vi "single sweep - next chunk - V2-2.vi"(4 "algorithm":string="statemachine", 5 "cursor bracket: Scan, win":refnum<vi>, 6 "mode":enum16{"first time", "uniform", "adaptive"}(ring)=enum."adaptive", 7 "Plot:response":refnum<vi>, 9 "x + iy":cdb[](array[numeric])=[0.0014961444378751654-0.005494848789731022i, 0.0014279223595474386-0.005470747752736027i, 0.001513711413730512-0.00552874878044623i, 0.001502407562898675-0.005445638194888334i, 0.0015845696982058808-0.005437153149732619i, 0.0015101628497750257-0.005522728337901211i, 0.0015131031857027845-0.005520920485579818i, 0.0015751707865244427-0.005432155579139866i, 0.001381283887581937-0.0055376532176146485i, 0.0013869914972504977-0.005471269712968517i], 10 "chunks":T1={"start F"=1400000.0, "stop F"=3000000.0, "total number of points"=6000, "chunk size"=10, "freq step (Hz)"=400.0, "update rate (Hz)"=250.0, "adaptive parameters"={"wavepacket"={"R"=0.5, "wave number"=15.0, "delta k"=7.0, "radii vector"=[], "radial section"=[], "wave vector"=22.0, "wavepacket is"=TRUE}, "number of grid points"=50, "decimation threshold"=1, "Voltage range"=0.1, "target freq step"=20.0, "target spot size"=0.05, "factor"=1.0, "another factor"=1.0, "analyze last # sec"=1, "scale factor"=10}, "total sweep time (sec)"=24.0, "chunk time (sec)"=0.04, "spot size (V)"=5.8152639158694506e-05, "uniform freq step (Hz)"=266.6666666666667, "next start freq"=1412960.0000000002} {"next start freq" format="%#_4f"; "uniform freq step (Hz)" format="%#_3f"; "spot size (V)" format="%#_2f"; "adaptive parameters"."wavepacket"."delta k" format="%#_3f"; "adaptive parameters"."wavepacket"."wave number" format="%#_3f"; "adaptive parameters"."wavepacket"."R" format="%#_3f"; "freq step (Hz)" format="%#_2f"; "stop F" format="%#_3f"; "start F" format="%#_3f"}, 11 "F Array in":dbl[](array[numeric])=[1408640.0000000002, 1408672.0000000002, 1408704.0000000002, 1408736.0000000002, 1408768.0000000002, 1408800.0000000002, 1408832.0000000002, 1408864.0000000002, 1408896.0000000002, 1408928.0000000002]) -> (0 "window":cluster{dbl[], dbl[]}[](array[cluster])=[{array[500 elements], array[500 elements]}, {array[500 elements], array[500 elements]}, {[2988000.0, 2988320.0, 2988640.0, 2992640.0, 2996640.0, 3000640.0, 3004640.0, 3004960.0, 3008960.0, 3012960.0, 3013280.0, 3013600.0, 3017600.0, 3021600.0, 3025600.0, 3029600.0, 3033600.0, 3037600.0, 3041600.0, 3045600.0, 3049600.0, 3053600.0, 3057600.0, 3061600.0, 3065600.0, 3069600.0, 3073600.0, 3077600.0, 3077920.0, 3081920.0, 3085920.0, 3089920.0, 3093920.0, 3094240.0, 3098240.0, 3102240.0, 3102560.0, 3106560.0, 3110560.0, 3114560.0, 3118560.0, 3122560.0, 3126560.0, 3126880.0, 3130880.0, 1408320.0000000002, 1408640.0000000002, 1408960.0000000002, 1412960.0000000002, 1416960.0000000002], [0.00011132389559019453, 0.00010071650784182846, 0.00011473215051580125, 0.00014782978553753255, 0.00012363182181742826, 8.247818640394286e-05, 4.853569183607435e-05, 0.00011091209952173231, 5.335161099533373e-05, 8.997863187674346e-05, 6.096859045620223e-05, 0.00011032129342938127, 0.00014137261844608594, 0.00011027777124700277, 7.83124094059187e-05, 8.359930932665522e-05, 8.923138939621333e-05, 5.1551353463386254e-05, 8.295869472945261e-05, 8.128556971740557e-05, 7.69462000730066e-05, 7.144851315975473e-05, 7.952519321081926e-05, 9.517779850815267e-05, 9.704248606160299e-05, 0.00011632633414436816, 0.00010390576558171027, 0.00010696411213824573, 9.728970607203878e-05, 0.0001308279684608251, 6.464132471543712e-05, 0.00011952708368690759, 6.148514772660781e-05, 8.068062707804084e-05, 0.00011312139911462234, 6.908047023895298e-05, 5.936822230667681e-05, 0.00010020626764101784, 0.00012946703718681504, 0.00010013466000813908, 6.912354981532708e-05, 0.00011430443059521424, 0.00012513022719631484, 0.00010923915541343698, 0.00011547570124367561, 0.003905008531492904, 0.0033917347983675613, 0.003353407371274829, 0.003173893478063239, 0.003074549188462509]}, {[2988000.0, 2988320.0, 2988640.0, 2992640.0, 2996640.0, 3000640.0, 3004640.0, 3004960.0, 3008960.0, 3012960.0, 3013280.0, 3013600.0, 3017600.0, 3021600.0, 3025600.0, 3029600.0, 3033600.0, 3037600.0, 3041600.0, 3045600.0, 3049600.0, 3053600.0, 3057600.0, 3061600.0, 3065600.0, 3069600.0, 3073600.0, 3077600.0, 3077920.0, 3081920.0, 3085920.0, 3089920.0, 3093920.0, 3094240.0, 3098240.0, 3102240.0, 3102560.0, 3106560.0, 3110560.0, 3114560.0, 3118560.0, 3122560.0, 3126560.0, 3126880.0, 3130880.0, 1408320.0000000002, 1408640.0000000002, 1408960.0000000002, 1412960.0000000002, 1416960.0000000002], [0.013694694005932529, 0.014489837272950239, 0.009503558469975002, 0.009528211653947193, 0.012476459558180022, 0.013578618032833986, 0.020768560303619083, 0.020949019291147796, 0.02034486055557658, 0.011646926818591538, 0.009458678658119484, 0.006310537358577627, 0.00038583342676350336, 0.006103250811137311, 0.001250242454873757, 0.005243640192020321, 0.008719705117003948, 0.006143859432854482, 0.006470257084291946, 0.006348276391260311, 0.008375758813583493, 0.0038044691071716097, 0.0015818509944146705, 0.003581191521982118, 0.0006892804064302445, 0.0025054554152808646, 0.004117073317010084, 0.002045540413627015, 0.0007410657254269008, 0.005324792655608368, 0.012491486267365477, 0.013829845176253889, 0.009382411909246033, 0.008531253899751555, 0.006057094794442862, 0.000802518050976467, 0.006846069080773061, 0.004537353265510852, 0.008159903085244793, 0.0028444703551188284, 0.007454427723095375, 4.4410190171195404e-05, 0.0015101954709487865, 0.004475681662266171, 0.010341490132182555, 0.01226244459723875, 0.015308020505903021, 0.005597683037877003, 0.0037965342629815418, 0.0016913227005998597]}], 1 "fancy circles":cluster{dbl[], dbl[]}[](array[cluster])=[{[0.004347976639836461, 0.0043237329011621035, 0.004251384023380436, 0.004132070991513198, 0.003967675443347089, 0.0037607899948818246, 0.0035146773532270816, 0.00323321886176232, 0.0029208532890330928, 0.002582506826719488, 0.00222351540065057, 0.0018495405200665291, 0.0014664799922359413, 0.001080374910511962, 0.0006973143826813736, 0.0003233395020973332, -3.56519239715844e-05, -0.0003739983862851902, -0.0006863639590144167, -0.0009678224504791784, -0.0012139350921339205, -0.0014208205405991845, -0.001585216088765295, -0.0017045291206325324, -0.0017768779984142003, -0.001801121737088557, -0.0017768779984142003, -0.0017045291206325324, -0.0015852160887652941, -0.001420820540599184, -0.00121393509213392, -0.000967822450479178, -0.0006863639590144162, -0.00037399838628518847, -3.5651923971582664e-05, 0.0003233395020973332, 0.0006973143826813741, 0.0010803749105119625, 0.0014664799922359426, 0.001849540520066531, 0.0022235154006505697, 0.002582506826719488, 0.0029208532890330936, 0.003233218861762321, 0.003514677353227083, 0.0037607899948818254, 0.003967675443347089, 0.004132070991513199, 0.004251384023380437, 0.0043237329011621035], [-0.00253283204245687, -0.0021474888509143563, -0.001768222751695333, -0.0014010149977470693, -0.0010516566747086093, -0.0007256573720308159, -0.00042815829345946126, -0.00016385117718095135, 6.309569569158376e-05, 0.0002491032374014545, 0.0003912379979003752, 0.0004872584271080889, 0.0005356502254961651, 0.0005356502254961651, 0.00048725842710808844, 0.0003912379979003752, 0.00024910323740145405, 6.309569569158376e-05, -0.00016385117718095135, -0.0004281582934594617, -0.0007256573720308154, -0.0010516566747086097, -0.00140101499774707, -0.0017682227516953328, -0.0021474888509143567, -0.002532832042456871, -0.002918175233999384, -0.003297441333218408, -0.003664649087166672, -0.004014007410205131, -0.004340006712882925, -0.004637505791454279, -0.004901812907732789, -0.005128759780605325, -0.005314767322315195, -0.005456902082814115, -0.0055529225120218295, -0.005601314310409906, -0.005601314310409906, -0.005552922512021829, -0.005456902082814115, -0.005314767322315195, -0.0051287597806053235, -0.004901812907732788, -0.004637505791454277, -0.004340006712882922, -0.004014007410205131, -0.0036646490871666704, -0.0032974413332184063, -0.0029181752339993822]}, {[-0.0007985969840225416, -0.0005913945404828922, -0.0003841920969432428, -0.0001769896534035934, 3.0212790136055923e-05, 0.00023741523367570524, 0.0004446176772153548, 0.0006518201207550041, 0.0008590225642946534, 0.0010662250078343027, 0.001273427451373952, 0.0014806298949136016, 0.001687832338453251, 0.0018950347819929002, 0.00210223722553255, 0.0023094396690721986, 0.002516642112611848, 0.0027238445561514977, 0.0029310469996911472, 0.003138249443230796], [-0.004804300169328853, -0.004577153356641655, -0.004350006543954456, -0.004122859731267258, -0.00389571291858006, -0.0036685661058928616, -0.003441419293205663, -0.003214272480518465, -0.0029871256678312666, -0.002759978855144068, -0.00253283204245687, -0.0023056852297696716, -0.002078538417082473, -0.0018513916043952751, -0.0016242447917080766, -0.0013970979790208786, -0.0011699511663336801, -0.0009428043536464817, -0.0007156575409592832, -0.0004885107282720852]}, {[-0.0009980406754980312, -0.0007708938628108329, -0.0005437470501236345, -0.0003166002374364362, -8.945342474923792e-05, 0.00013769338793796033, 0.0003648402006251588, 0.0005919870133123571, 0.0008191338259995553, 0.0010462806386867538, 0.0012734274513739518, 0.0015005742640611503, 0.0017277210767483488, 0.001954867889435547, 0.0021820147021227453, 0.0024091615148099433, 0.002636308327497142, 0.0028634551401843403, 0.0030906019528715387, 0.0033177487655587368], [-0.0004608076070603765, -0.0006680100506000258, -0.0008752124941396752, -0.0010824149376793247, -0.001289617381218974, -0.0014968198247586233, -0.0017040222682982728, -0.0019112247118379222, -0.0021184271553775715, -0.0023256295989172206, -0.00253283204245687, -0.0027400344859965196, -0.002947236929536169, -0.0031544393730758183, -0.003361641816615468, -0.003568844260155117, -0.0037760467036947664, -0.003983249147234416, -0.004190451590774065, -0.004397654034313714]}], 2 "chunks out":T1={"start F"=1400000.0, "stop F"=3000000.0, "total number of points"=6000, "chunk size"=10, "freq step (Hz)"=400.0, "update rate (Hz)"=250.0, "adaptive parameters"={"wavepacket"={"R"=0.5, "wave number"=15.0, "delta k"=7.0, "radii vector"=[], "radial section"=[], "wave vector"=22.0, "wavepacket is"=TRUE}, "number of grid points"=50, "decimation threshold"=1, "Voltage range"=0.1, "target freq step"=20.0, "target spot size"=0.05, "factor"=1.0, "another factor"=1.0, "analyze last # sec"=1, "scale factor"=10}, "total sweep time (sec)"=24.0, "chunk time (sec)"=0.04, "spot size (V)"=5.8152639158694506e-05, "uniform freq step (Hz)"=266.6666666666667, "next start freq"=1412960.0000000002} {"next start freq" format="%#_4f"; "uniform freq step (Hz)" format="%#_3f"; "spot size (V)" format="%#_2f"; "adaptive parameters"."wavepacket"."delta k" format="%#_3f"; "adaptive parameters"."wavepacket"."wave number" format="%#_3f"; "adaptive parameters"."wavepacket"."R" format="%#_3f"; "freq step (Hz)" format="%#_2f"; "stop F" format="%#_3f"; "start F" format="%#_3f"}, 3 "F Array":dbl[](array[numeric])=[1412960.0000000002, 1413360.0000000002, 1413760.0000000002, 1414160.0000000002, 1414560.0000000002, 1414960.0000000002, 1415360.0000000002, 1415760.0000000002, 1416160.0000000002, 1416560.0000000002])   [LabVIEW 2010]
uses:
  single sweep - frequency chunks.ctl
  single sweep - adaptive parameters.ctl
  wavepacket.ctl
  generate wave packet V2.vi
  smart decimate .vi
  set up complex region.vi
  inteference -- find center V2.vi
  find circle corners V3.vi
  peak - phase around center.vi
  peak - simple guess at omega.vi
  peak - fix phase.vi
  peak - fit phase around center.vi
  peak - calculate lorentzian.vi
  draw a line.vi
  draw a circle.vi
  generate linear region.vi
  find circle corners - rescale back.vi
  <vilib>/Analysis/baseanly.llb/Median.vi
  <vilib>/Analysis/baseanly.llb/Mean.vi
  <vilib>/Analysis/2dsp.llb/Unwrap Phase.vi
  <vilib>/gmath/NumericalOptimization/Nonlinear Curve Fit.vi
  <vilib>/gmath/NumericalOptimization/Nonlinear Curve Fit LM.vi
  <vilib>/Utility/error.llb/Clear Errors.vi
panel:
  in  "search win (kHz)":dbl=12.0
  in  "scale factor":i32=3
  out "viscosity":dbl
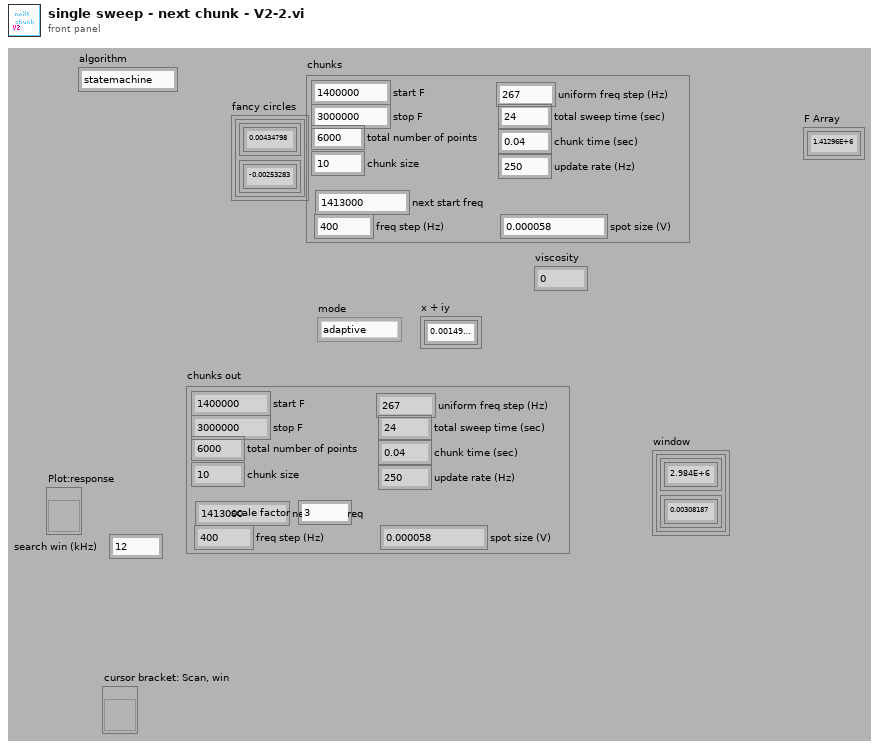
[diagram p1: front panel]
types:
  T1 = typedef "single sweep - frequency chunks.ctl" = cluster{"start F":dbl, "stop F":dbl, "total number of points":i32, "chunk size":i32, "freq step (Hz)":dbl, "update rate (Hz)":dbl, "adaptive parameters":T2, "total sweep time (sec)":dbl, "chunk time (sec)":dbl, "spot size (V)":dbl, "uniform freq step (Hz)":dbl, "next start freq":dbl}
  T2 = typedef "single sweep - adaptive parameters.ctl" = cluster{"wavepacket":T3, "number of grid points":i32, "decimation threshold":i32, "Voltage range":dbl, "target freq step":dbl, "target spot size":dbl, "factor":dbl, "another factor":dbl, "analyze last # sec":i32, "scale factor":i32}
  T3 = typedef "wavepacket.ctl" = cluster{"R":dbl, "wave number":dbl, "delta k":dbl, "radii vector":dbl[], "radial section":cdb[], "wave vector":dbl, "wavepacket is":bool}
  T4 = enum16{"", "cursor moves", "center change", "window change", "init", "check", "reset", "set y to middle"}
  T5 = typedef "circle corners.ctl" = cluster{"z (-pi/2)":cdb, "z(inf)":cdb, "z (pi/2)":cdb, "z center":cdb, "z(0)":cdb, "radius":dbl}
  T6 = typedef "lorentzian.ctl" = cluster{"Amplitude":dbl, "omega(0)":dbl, "Gamma":dbl, "phase":dbl, "Q":dbl, "Norm  Ampl":dbl, "z (inf)":cdb, "4corners":T5}
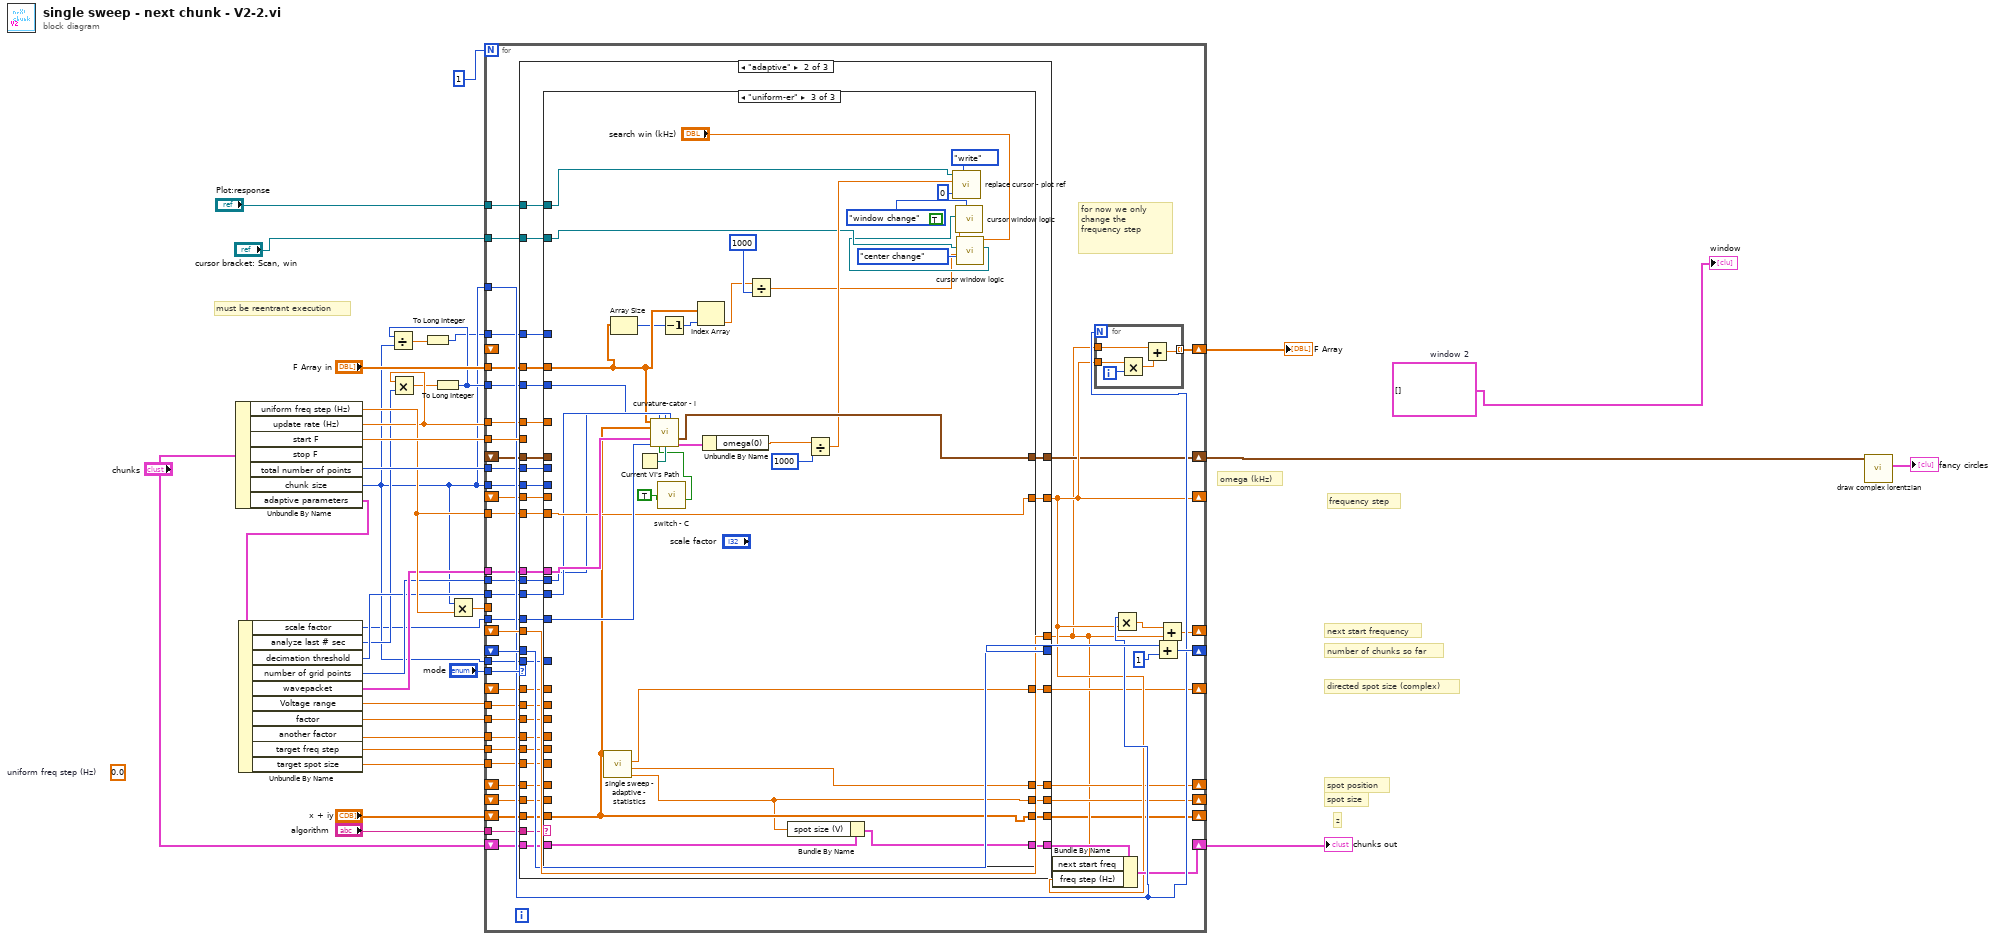
[diagram p0: block diagram]
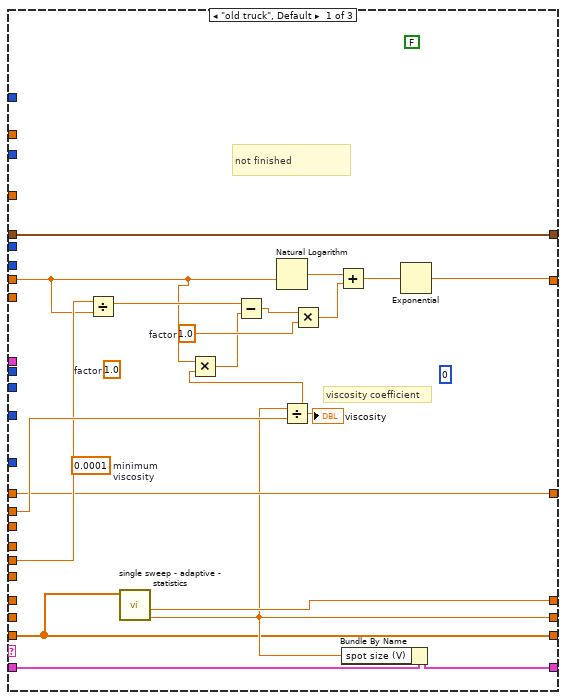
[diagram p3: hidden frame]
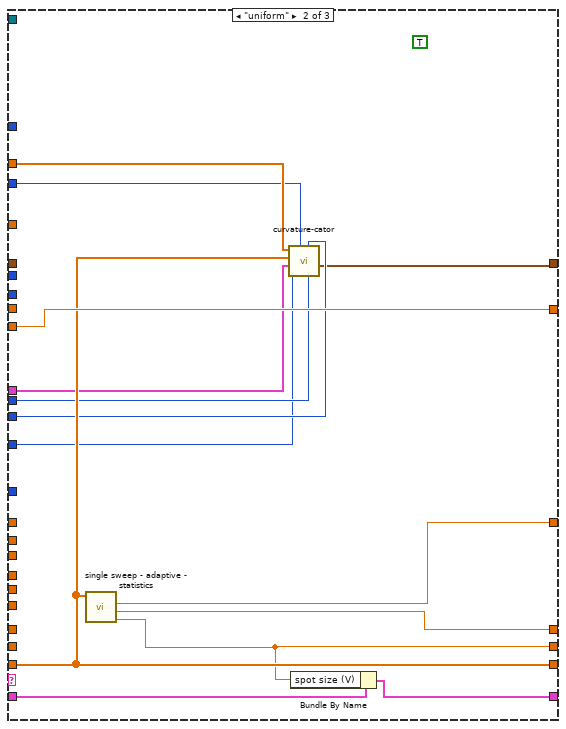
[diagram p4: hidden frame]
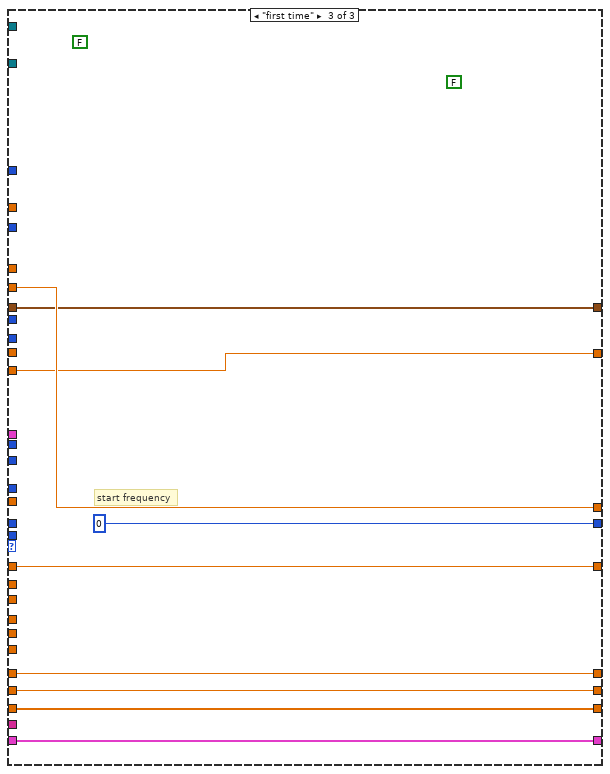
[diagram p5: hidden frame]
diagram:
  w1 = cluster{dbl[], dbl[]}[] []  # window 2
  (unwired) 0.0  # uniform freq step (Hz)
  # "omega (kHz)"
  # "z"
  # "must be reentrant execution"
  # "directed spot size (complex)"
  # "spot position"
  # "spot size"
  # "frequency step"
  # "number of chunks so far"
  # "next start frequency"
  n1 = Unbundle By Name("chunks") -> ("uniform freq step (Hz)"=w19:dbl, "update rate (Hz)"=w17:dbl, "start F"=w32:dbl, "total number of points"=w28:i32, "chunk size"=w9:i32, "adaptive parameters"=w25:T2)  [unwired: 1 out]
  n2 = Unbundle By Name(w25) -> ("scale factor"=w4:i32, "analyze last # sec"=w13:i32, "decimation threshold"=w14:i32, "number of grid points"=w15:i32, "wavepacket"=w16:T3, "Voltage range"=w21:dbl, "factor"=w23:dbl, "another factor"=w22:dbl, "target freq step"=w24:dbl, "target spot size"=w20:dbl)
  n3 = Multiply(x=w17, y=w13) -> (x*y=w12:dbl)
  n4 = To Long Integer(number=w12) -> (32bit integer=w10:i32)
  n5 = Divide(x=w10, y=w9) -> (x/y=w8:dbl)
  n6 = To Long Integer(number=w8) -> (32bit integer=w7:i32)
  n7 = Multiply(x=w9, y=w19) -> (x*y=w33:dbl)
  n8 = for {
    N: 1 -> [_]
    tunnel: w19 -> [w51]
    tunnel: w9 -> [w73]
    tunnel: "mode" -> [w81]
    shift-right: [w41] -> _
    shift-left: _ -> [w79]
    shift-right: [w76] -> _
    shift-left: _ -> [w78]
    tunnel: w33 -> [_]
    tunnel: w32 -> [w74]
    shift-right: [w80] -> w11
    shift-left: _ -> [_]
    tunnel: "F Array in" -> [w70]
    tunnel: w9 -> [w69]
    tunnel: w28 -> [w68]
    tunnel: w21 -> [w67]
    shift-right: [w66] -> w27
    shift-left: "chunks" -> [w61]
    shift-right: [w65] -> _
    shift-left: _ -> [w64]
    tunnel: "algorithm" -> [w63]
    tunnel: w24 -> [w62]
    shift-right: [w59] -> _
    shift-left: _ -> [w56]
    shift-right: [w58] -> _
    shift-left: _ -> [w57]
    tunnel: w9 -> [w55]
    shift-right: [w54] -> _
    shift-left: _ -> [w52]
    tunnel: w20 -> [w53]
    tunnel: w23 -> [w50]
    tunnel: w22 -> [w49]
    tunnel: w17 -> [w48]
    tunnel: w10 -> [w47]
    tunnel: w16 -> [w46]
    tunnel: w15 -> [w45]
    tunnel: w14 -> [w44]
    shift-right: [w43] -> w5
    shift-left: _ -> [w42]
    shift-right: [w39] -> _
    shift-left: "x + iy" -> [w71]
    tunnel: w7 -> [w38]
    tunnel: w4 -> [w37]
    tunnel: "cursor bracket: Scan, win" -> [w36]
    tunnel: "Plot:response" -> [w35]
    # "for now we only change the \nfrequency step"
    n9 = case shown="\"adaptive\"" w81 {
      tunnel: [w90 w126 w201] -> w40
      tunnel: [w88 w125 0] -> w77
      tunnel: w79 -> [w90 w126 _]
      tunnel: w78 -> [w88 w125 _]
      tunnel: w74 -> [_ _ w201]
      tunnel: [w89 w123 w196] -> w65
      tunnel: w64 -> [w89 w124 _]
      tunnel: w71 -> [w82 w122 w194]
      tunnel: w70 -> [_ w121 _]
      tunnel: w69 -> [_ w120 _]
      tunnel: w68 -> [_ w119 _]
      tunnel: w67 -> [_ w118 _]
      tunnel: w63 -> [_ w117 _]
      tunnel: w62 -> [_ w116 _]
      tunnel: w61 -> [w87 w115 w200]
      tunnel: [w87 w114 w200] -> w60
      tunnel: [w85 w113 w198] -> w59
      tunnel: [w86 w112 w199] -> w58
      tunnel: w57 -> [w86 w111 w199]
      tunnel: w56 -> [w85 w110 w198]
      tunnel: w55 -> [_ w109 _]
      tunnel: [w84 w108 w197] -> w54
      tunnel: w53 -> [_ w107 _]
      tunnel: w52 -> [w84 w106 w197]
      tunnel: w51 -> [_ w103 w196]
      tunnel: w50 -> [_ w105 _]
      tunnel: w49 -> [_ w104 _]
      tunnel: w48 -> [_ w102 _]
      tunnel: w47 -> [_ w101 _]
      tunnel: w46 -> [_ w100 _]
      tunnel: w45 -> [_ w99 _]
      tunnel: w44 -> [_ w98 _]
      tunnel: [w83 w97 w195] -> w43
      tunnel: w42 -> [w83 w96 w195]
      tunnel: [w82 w95 w194] -> w39
      tunnel: w38 -> [_ w94 _]
      tunnel: w37 -> [_ w93 _]
      tunnel: w36 -> [_ w92 _]
      tunnel: w35 -> [_ w91 _]
      frame "uniform" {
        # "keep frequency step constant,  as determined by global values"
      }
      frame "adaptive" {
        n10 = case shown="\"uniform-er\"" w117 {
          tunnel: w124 -> [w132 _ _]
          tunnel: [w135 w159 w178] -> w123
          tunnel: w122 -> [w127 w155 w163]
          tunnel: w121 -> [_ w156 w170]
          tunnel: w120 -> [_ _ _]
          tunnel: w119 -> [_ _ _]
          tunnel: w118 -> [w141 _ _]
          tunnel: w116 -> [w140 _ _]
          tunnel: w115 -> [w143 w147 w165]
          tunnel: [w142 w148 w164] -> w114
          tunnel: [w129 w149 w160] -> w113
          tunnel: [w130 w158 w161] -> w112
          tunnel: w111 -> [_ _ _]
          tunnel: w110 -> [_ _ _]
          tunnel: w109 -> [_ _ _]
          tunnel: [w131 w157 w162] -> w108
          tunnel: w107 -> [_ _ _]
          tunnel: w106 -> [w131 _ _]
          tunnel: w105 -> [_ _ _]
          tunnel: w104 -> [_ _ _]
          tunnel: w103 -> [_ w159 w178]
          tunnel: w102 -> [_ _ _]
          tunnel: w101 -> [_ w151 w173]
          tunnel: w100 -> [_ w154 w184]
          tunnel: w99 -> [_ w152 w174]
          tunnel: w98 -> [_ w153 w175]
          tunnel: [w128 w150 w179] -> w97
          tunnel: w96 -> [w128 _ _]
          tunnel: [w127 w155 w163] -> w95
          tunnel: w94 -> [_ _ _]
          tunnel: w93 -> [_ w146 w180]
          tunnel: w92 -> [_ _ w172]
          tunnel: w91 -> [_ _ w176]
          frame "old truck", Default {
            (unwired) 0
            (unwired) FALSE
            (unwired) 1.0  # factor
            w138 = 1.0  # factor
            (unwired) 0.0001  # minimum  viscosity
            # "not finished"
            # "viscosity coefficient"
            n11 = Divide(x=w140, y=w132) -> (x/y=w139:dbl)
            n12 = call "single sweep - adaptive - statistics.vi"("x + iy"=w127) -> ("spot size"=w129:dbl, "spot position"=w130:cdb)  [unwired: 8 in, 1 out]
            n13 = Natural Logarithm(1:w132) -> (0:w137:dbl)
            n14 = Divide(x=w129, y=w141) -> (x/y=w134:dbl)
            "viscosity" <- w134
            n15 = Multiply(x=w132, y=w134) -> (x*y=w133:dbl)
            n16 = Subtract(x=w139, y=w133) -> (x-y=w145:dbl)
            n17 = Multiply(x=w145, y=w138) -> (x*y=w144:dbl)
            n18 = Add(x=w137, y=w144) -> (x+y=w136:dbl)
            n19 = Bundle By Name(cluster=w143, "spot size (V)"=w129) -> (w142:T1)
            n20 = Exponential(1:w136) -> (0:w135:dbl)
          }
          frame "uniform" {
            (unwired) TRUE
            n21 = call "single sweep - adaptive - statistics.vi"("x + iy"=w155) -> ("spot size"=w149:dbl, "spot position"=w158:cdb, "spot directed size"=w157:cdb)  [unwired: 8 in]
            n22 = call "curvature-cator.vi"("number of grid points"=w152, "decimation threshold"=w153, "size"=w151, "scale factor"=w146, "wavepacket in"=w154, "z array in"=w155, "omega array in"=w156) -> ("4 corners out"=w150:T5)  [unwired: 2 in, 2 out]
            n23 = Bundle By Name(cluster=w147, "spot size (V)"=w149) -> (w148:T1)
          }
          frame "uniform-er" {
            (unwired) TRUE
            n24 = call "single sweep - adaptive - statistics.vi"("x + iy"=w163) -> ("spot size"=w160:dbl, "spot position"=w161:cdb, "spot directed size"=w162:cdb)  [unwired: 8 in]
            n25 = Array Size(array=w170) -> (size(s)=w169:i32)
            n26 = Current VI's Path() -> (path=w193:path)
            n27 = call "switch - C.vi"("switch"=TRUE) -> ("result"=w183:bool)  [unwired: 10 in]
            n28 = call "curvature-cator - i.vi"("omega array in"=w170, "size"=w173, "number of grid points"=w174, "decimation threshold"=w175, "z array in"=w163, "wavepacket in"=w184, "scale factor"=w180, "first time"=w183, "main VI path"=w193) -> ("4 corners rescaled out"=w179:T5, "lorentzian out"=w192:T6)  [unwired: 3 in, 2 out]
            n29 = Decrement(x=w169) -> (x-1=w186:i32)
            n30 = Index Array(array=w170, index=w186) -> (element=w168:dbl)
            n31 = Unbundle By Name(w192) -> ("omega(0)"=w182:dbl)
            n32 = Divide(x=w168, y=1000) -> (x/y=w167:dbl)
            n33 = Bundle By Name(cluster=w165, "spot size (V)"=w160) -> (w164:T1)
            n34 = Divide(x=w182, y=1000) -> (x/y=w177:dbl)
            n35 = call "replace cursor - plot ref.vi"("action"=enum16{"", "read", "write"}."write", "cursor index"=0, "new X"=w177, "Plot ref in"=w176) -> ()  [unwired: 5 in, 3 out]
            n36 = call "cursor window logic.vi"("action"=T4."center change", "center"=w167, "cursor bracket in"=w172) -> ("cursor bracket out"=w171:refnum<vi>)  [unwired: 7 in, 1 out]
            n37 = call "cursor window logic.vi"("action"=T4."window change", "window"="search win (kHz)", "cursor bracket in"=w171) -> ()  [unwired: 7 in, 2 out]
          }
        }
      }
      frame "first time" {
        (unwired) FALSE
        (unwired) FALSE
        # "start frequency"
      }
    }
    n38 = Bundle By Name(cluster=w60, "next start freq"=w40, "freq step (Hz)"=w65) -> (w66:T1)
    n39 = for {
      N: w73 -> [_]
      tunnel: w65 -> [w207]
      tunnel: [w205] -> w80 mode=indexing
      tunnel: w40 -> [w203]
      i -> [w204]
      n40 = Multiply(x=w207, y=w204) -> (x*y=w206:dbl)
      n41 = Add(x=w203, y=w206) -> (x+y=w205:dbl)
    }
    n42 = Multiply(x=w73, y=w65) -> (x*y=w72:dbl)
    n43 = Add(x=w77, y=1) -> (x+y=w76:i32)
    n44 = Add(x=w72, y=w40) -> (x+y=w41:dbl)
  }
  "F Array" <- w11
  "chunks out" <- w27
  n45 = call "draw complex lorentzian.vi"("4 corners"=w5) -> ("fancy circles"=→"fancy circles":cluster{dbl[], dbl[]}[])  [unwired: 10 in]
  "window" <- w1
